vi "AutoIncrement Version String.vi"(8 "error in":errorcluster, 11 "Version String":string="1.0.0") -> (0 "error out":errorcluster, 3 "AutoIncrement String":string)   [LabVIEW 2023]
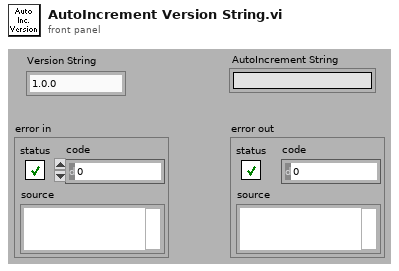
[diagram p1: front panel]
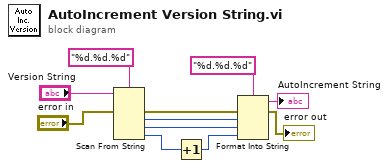
[diagram p0: block diagram]
diagram:
  n1 = Scan From String(format string="%d.%d.%d", input string="Version String", error in="error in") -> (error out=w2:errorcluster, output 1=w6:i32, output 2=w5:i32, output 3=w10:i32)  [unwired: 4 in, 2 out]
  n2 = Increment(x=w10) -> (x+1=w7:i32)
  n3 = Format Into String(format string="%d.%d.%d", error in=w2, w6, w5, w7) -> (resulting string=→"AutoIncrement String":string, error out=→"error out":errorcluster)  [unwired: 1 in]
